vi "getDeviceType.vi"(8 "error in (no error)":errorcluster, 11 "RfOutputData in":refnum<class "RfOutputData.lvclass">) -> (0 "error out":errorcluster, 2 "type":T1(ring), 3 "RfOutputData out":refnum<class "RfOutputData.lvclass">)   [LabVIEW 2011, in "DataMappers.lvlib" / "RfOutputData.lvclass"]
uses:
  RfOutputData.lvclass
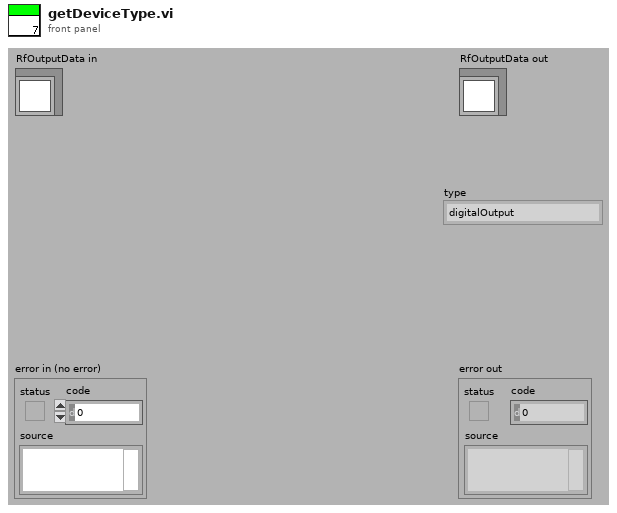
[diagram p1: front panel]
types:
  T1 = enum16{"digitalOutput", "digitalInput", "analogOutput", "analogInput", "rfOutput", "ethernetSupply"}
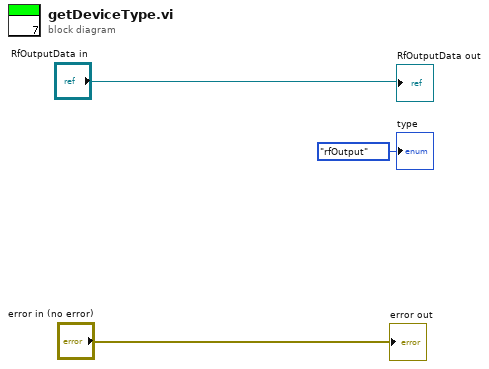
[diagram p0: block diagram]
diagram:
  "error out" <- "error in (no error)"
  "RfOutputData out" <- "RfOutputData in"
  "type" <- T1."rfOutput" ("type")
